vi "KE2260B Output Protection Tripped.vi"(8 "error in (no error)":errorcluster, 11 "VISA resource name":refnum<visa-resource-name>) -> (0 "error out":errorcluster, 1 "OCP Tripped?":bool, 2 "OVP Tripped?":bool, 3 "VISA resource name out":refnum<visa-resource-name>, 4 "OTP Tripped?":bool, 5 "AC Power Off?":bool, 6 "Shutdown Tripped?":bool, 7 "Protection Tripped?":bool)   [LabVIEW 2009, in "Keithley 2260B.lvlib"]
doc: "Returns TRUE if the protection circuit (over-voltage or over-current or over-temperature or shutdown or AC failure) is tripped and a FALSE if it is untripped."
uses:
  <instrlib>/Keithley 2260B/Keithley 2260B.lvlib
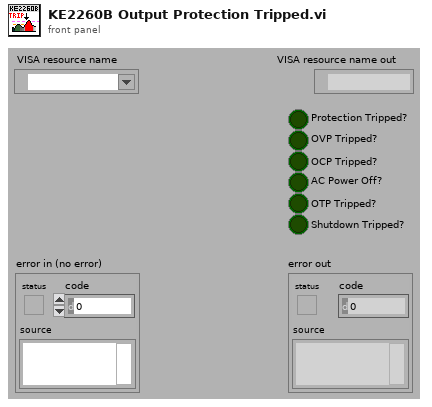
[diagram p1: front panel]
types:
  T1 = cluster{"Boolean array[0]":bool, "Boolean array[1]":bool, "Boolean array[2]":bool, "Boolean array[3]":bool, "Boolean array[4]":bool, "Boolean array[5]":bool, "Boolean array[6]":bool, "Boolean array[7]":bool, "Boolean array[8]":bool, "Boolean array[9]":bool, "Boolean array[10]":bool, "Boolean array[11]":bool, "Boolean array[12]":bool, "Boolean array[13]":bool, "Boolean array[14]":bool, "Boolean array[15]":bool}
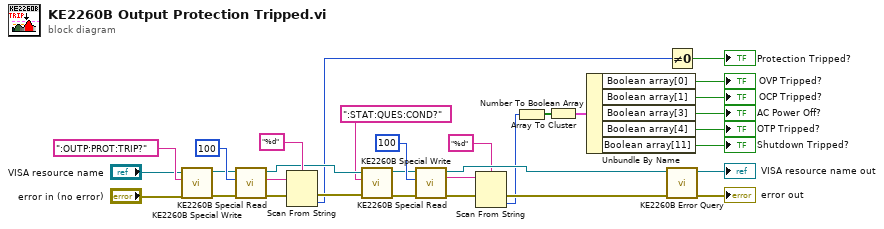
[diagram p0: block diagram]
diagram:
  n1 = call <instrlib>:"KE2260B Special Write.vi"("error in (no error)"="error in (no error)", "Write Buffer (\"\")"=":OUTP:PROT:TRIP?" ("write buffer"), "VISA session"="VISA resource name") -> ("error out"=w27:errorcluster, "dup VISA session"=w25:refnum<visa-resource-name>)  [unwired: 6 in, 1 out]
  n2 = call <instrlib>:"KE2260B Special Read.vi"("error in (no error)"=w27, "byte count"=u32 100, "VISA session"=w25) -> ("error out"=w21:errorcluster, "read buffer"=w20:string, "dup VISA session"=w19:refnum<visa-resource-name>)  [unwired: 5 in, 1 out]
  n3 = Scan From String(format string="%d", input string=w20, error in=w21) -> (error out=w18:errorcluster, output 1=w1:i32)  [unwired: 2 in, 2 out]
  n4 = call <instrlib>:"KE2260B Special Write.vi"("error in (no error)"=w18, "Write Buffer (\"\")"=":STAT:QUES:COND?" ("write buffer"), "VISA session"=w19) -> ("error out"=w8:errorcluster, "dup VISA session"=w6:refnum<visa-resource-name>)  [unwired: 6 in, 1 out]
  n5 = call <instrlib>:"KE2260B Special Read.vi"("error in (no error)"=w8, "byte count"=u32 100, "VISA session"=w6) -> ("error out"=w9:errorcluster, "read buffer"=w11:string, "dup VISA session"=w29:refnum<visa-resource-name>)  [unwired: 5 in, 1 out]
  n6 = Scan From String(format string="%d", input string=w11, error in=w9) -> (error out=w30:errorcluster, output 1=w5:i32)  [unwired: 2 in, 2 out]
  n7 = Number To Boolean Array(number=w5) -> (Boolean array=w4:bool[])
  n8 = Array To Cluster(array=w4) -> (cluster=w3:T1)
  n9 = Unbundle By Name(w3) -> ("Boolean array[0]"=→"OVP Tripped?":bool, "Boolean array[1]"=→"OCP Tripped?":bool, "Boolean array[3]"=→"AC Power Off?":bool, "Boolean array[4]"=→"OTP Tripped?":bool, "Boolean array[11]"=→"Shutdown Tripped?":bool)
  n10 = Not Equal To 0?(x=w1) -> (x != 0?=→"Protection Tripped?":bool)
  n11 = call <instrlib>:"KE2260B Error Query.vi"("error in (no error)"=w30, "VISA resource name"=w29) -> ("error out"=→"error out":errorcluster, "VISA resource name out"=→"VISA resource name out":refnum<visa-resource-name>)  [unwired: 6 in, 2 out]
